vi "prop_axes_page_to_prop.vi"(10 "Axes Property Page":T1(array[cluster])) -> (2 "Axes Properties Out":T2)   [LabVIEW 2020, in "3DPC_SurfacePlot.xctl"]
uses:
  <vilib>/Native 3D Graph/xcontrol/3DPC_SurfacePlot.xctl
  <vilib>/Native 3D Graph/typedefs/prop_axes_all.ctl
  <vilib>/Native 3D Graph/typedefs/prop_axes_grid.ctl
  <vilib>/Native 3D Graph/typedefs/prop_axes_ticks.ctl
  <vilib>/Native 3D Graph/typedefs/range_cluster.ctl
  <vilib>/Native 3D Graph/typedefs/min_max.ctl
  <vilib>/Native 3D Graph/typedefs/prop_axes_captions.ctl
  <vilib>/Native 3D Graph/typedefs/prop_axes_labels.ctl
  <vilib>/Native 3D Graph/typedefs/prop_axes_autorange.ctl
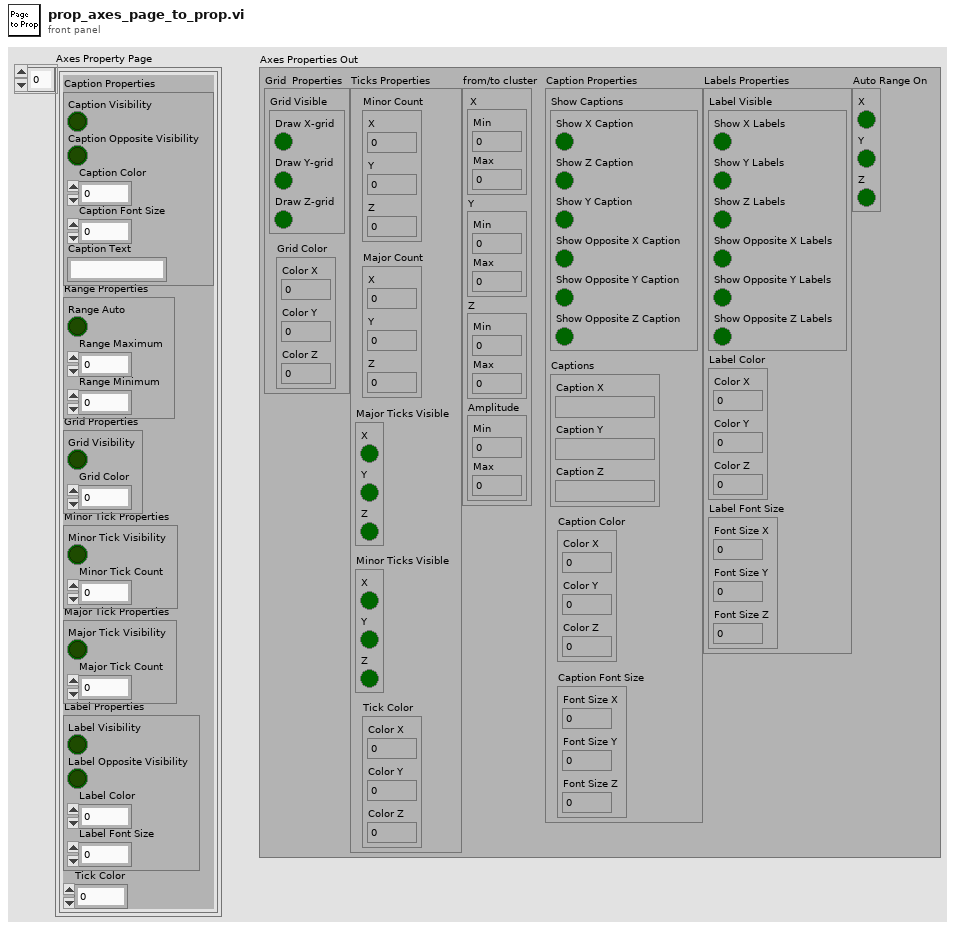
[diagram p1: front panel]
types:
  T1 = cluster{"Caption Properties":cluster{"Caption Visibility":bool, "Caption Opposite Visibility":bool, "Caption Color":u32, "Caption Font Size":i32, "Caption Text":string}, "Range Properties":cluster{"Range Auto":bool, "Range Maximum":dbl, "Range Minimum":dbl}, "Grid Properties":cluster{"Grid Visibility":bool, "Grid Color":u32}, "Minor Tick Properties":cluster{"Minor Tick Visibility":bool, "Minor Tick Count":i32}, "Major Tick Properties":cluster{"Major Tick Visibility":bool, "Major Tick Count":i32}, "Label Properties":cluster{"Label Visibility":bool, "Label Opposite Visibility":bool, "Label Color":u32, "Label Font Size":i32}, "Tick Color":u32}[]
  T2 = typedef "3DPC_SurfacePlot.xctl/prop_axes_all.ctl" = cluster{"Grid  Properties":T3, "Ticks Properties":T4, "from/to cluster":T5, "Caption Properties":T7, "Labels Properties":T8, "Auto Range On":T9}
  T3 = typedef "3DPC_SurfacePlot.xctl/prop_axes_grid.ctl" = cluster{"Grid Visible":cluster{"Draw X-grid":bool, "Draw Y-grid":bool, "Draw Z-grid":bool}, "Grid Color":cluster{"Color X":u32, "Color Y":u32, "Color Z":u32}}
  T4 = typedef "3DPC_SurfacePlot.xctl/prop_axes_ticks.ctl" = cluster{"Minor Count":cluster{"X":i32, "Y":i32, "Z":i32}, "Major Count":cluster{"X":i32, "Y":i32, "Z":i32}, "Major Ticks Visible":cluster{"X":bool, "Y":bool, "Z":bool}, "Minor Ticks Visible":cluster{"X":bool, "Y":bool, "Z":bool}, "Tick Color":cluster{"Color X":u32, "Color Y":u32, "Color Z":u32}}
  T5 = typedef "3DPC_SurfacePlot.xctl/range_cluster.ctl" = cluster{"X":T6, "Y":T6, "Z":T6, "Amplitude":T6}
  T6 = typedef "3DPC_SurfacePlot.xctl/min_max.ctl" = cluster{"Min":sgl, "Max":sgl}
  T7 = typedef "3DPC_SurfacePlot.xctl/prop_axes_captions.ctl" = cluster{"Show Captions":cluster{"Show X Caption":bool, "Show Z Caption":bool, "Show Y Caption":bool, "Show Opposite X Caption":bool, "Show Opposite Y Caption":bool, "Show Opposite Z Caption":bool}, "Captions":cluster{"Caption X":string, "Caption Y":string, "Caption Z":string}, "Caption Color":cluster{"Color X":u32, "Color Y":u32, "Color Z":u32}, "Caption Font Size":cluster{"Font Size X":i16, "Font Size Y":i16, "Font Size Z":i16}}
  T8 = typedef "3DPC_SurfacePlot.xctl/prop_axes_labels.ctl" = cluster{"Label Visible":cluster{"Show X Labels":bool, "Show Y Labels":bool, "Show Z Labels":bool, "Show Opposite X Labels":bool, "Show Opposite Y Labels":bool, "Show Opposite Z Labels":bool}, "Label Color":cluster{"Color X":u32, "Color Y":u32, "Color Z":u32}, "Label Font Size":cluster{"Font Size X":i16, "Font Size Y":i16, "Font Size Z":i16}}
  T9 = typedef "3DPC_SurfacePlot.xctl/prop_axes_autorange.ctl" = cluster{"X":bool, "Y":bool, "Z":bool}
  T10 = cluster{"Caption Properties":cluster{"Caption Visibility":bool, "Caption Opposite Visibility":bool, "Caption Color":u32, "Caption Font Size":i32, "Caption Text":string}, "Range Properties":cluster{"Range Auto":bool, "Range Maximum":dbl, "Range Minimum":dbl}, "Grid Properties":cluster{"Grid Visibility":bool, "Grid Color":u32}, "Minor Tick Properties":cluster{"Minor Tick Visibility":bool, "Minor Tick Count":i32}, "Major Tick Properties":cluster{"Major Tick Visibility":bool, "Major Tick Count":i32}, "Label Properties":cluster{"Label Visibility":bool, "Label Opposite Visibility":bool, "Label Color":u32, "Label Font Size":i32}, "Tick Color":u32}
  T11 = cluster{"Range Minimum":dbl, "Range Maximum":dbl}
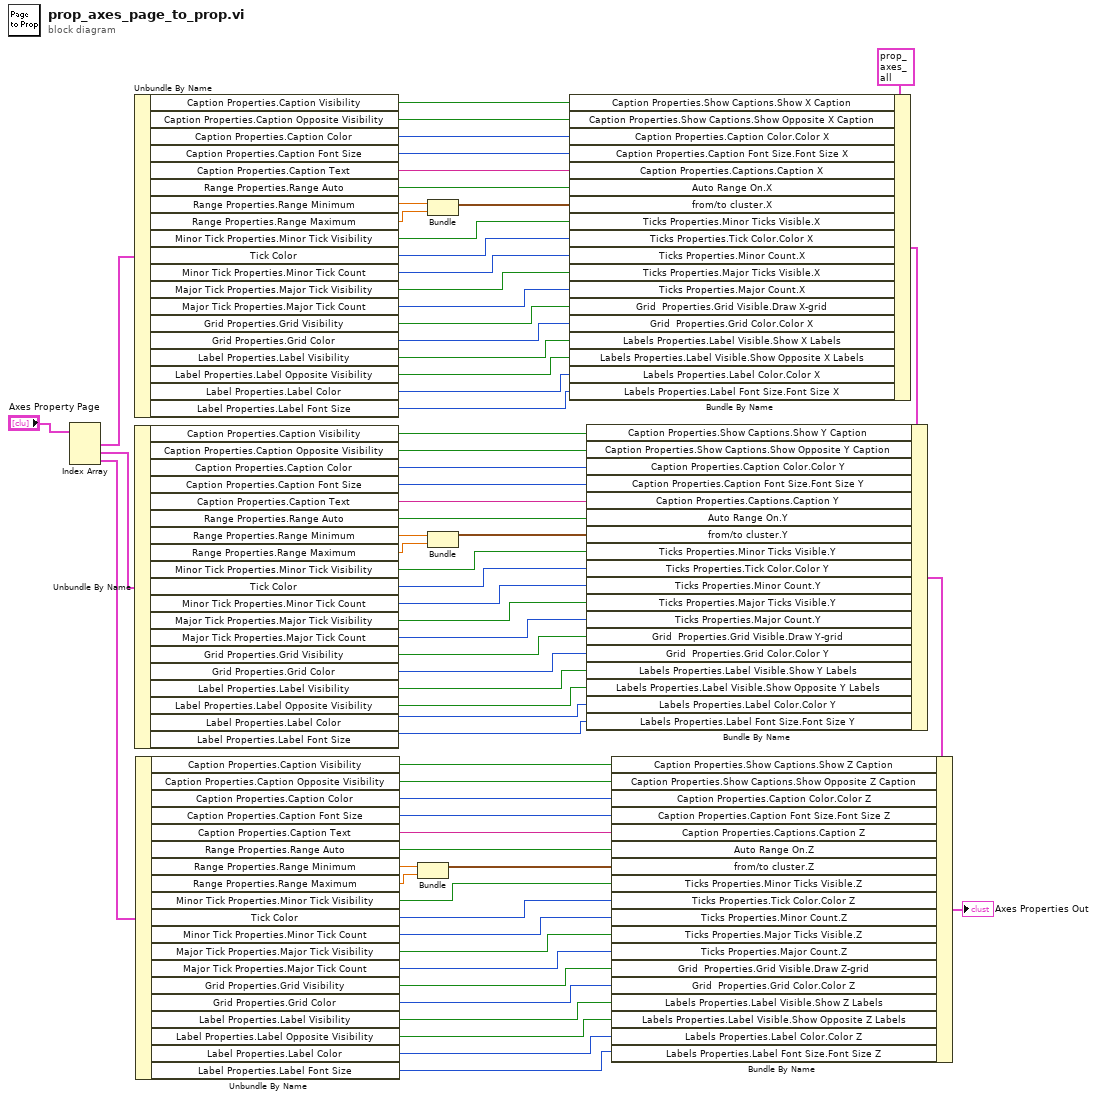
[diagram p0: block diagram]
diagram:
  n1 = Index Array(array="Axes Property Page") -> (element #1=w68:T10, element #2=w67:T10, element #3=w66:T10)  [unwired: 3 in]
  n2 = Unbundle By Name(w68) -> ("Caption Properties.Caption Visibility"=w58:bool, "Caption Properties.Caption Opposite Visibility"=w9:bool, "Caption Properties.Caption Color"=w57:u32, "Caption Properties.Caption Font Size"=w56:i32, "Caption Properties.Caption Text"=w55:string, "Range Properties.Range Auto"=w44:bool, "Range Properties.Range Minimum"=w65:dbl, "Range Properties.Range Maximum"=w64:dbl, "Minor Tick Properties.Minor Tick Visibility"=w54:bool, "Tick Color"=w53:u32, "Minor Tick Properties.Minor Tick Count"=w52:i32, "Major Tick Properties.Major Tick Visibility"=w51:bool, "Major Tick Properties.Major Tick Count"=w50:i32, "Grid Properties.Grid Visibility"=w49:bool, "Grid Properties.Grid Color"=w48:u32, "Label Properties.Label Visibility"=w47:bool, "Label Properties.Label Opposite Visibility"=w46:bool, "Label Properties.Label Color"=w45:u32, "Label Properties.Label Font Size"=w6:i32)
  n3 = Unbundle By Name(w67) -> ("Caption Properties.Caption Visibility"=w43:bool, "Caption Properties.Caption Opposite Visibility"=w8:bool, "Caption Properties.Caption Color"=w42:u32, "Caption Properties.Caption Font Size"=w41:i32, "Caption Properties.Caption Text"=w40:string, "Range Properties.Range Auto"=w39:bool, "Range Properties.Range Minimum"=w60:dbl, "Range Properties.Range Maximum"=w59:dbl, "Minor Tick Properties.Minor Tick Visibility"=w37:bool, "Tick Color"=w36:u32, "Minor Tick Properties.Minor Tick Count"=w35:i32, "Major Tick Properties.Major Tick Visibility"=w34:bool, "Major Tick Properties.Major Tick Count"=w33:i32, "Grid Properties.Grid Visibility"=w31:bool, "Grid Properties.Grid Color"=w30:u32, "Label Properties.Label Visibility"=w29:bool, "Label Properties.Label Opposite Visibility"=w28:bool, "Label Properties.Label Color"=w27:u32, "Label Properties.Label Font Size"=w5:i32)
  n4 = Unbundle By Name(w66) -> ("Caption Properties.Caption Visibility"=w25:bool, "Caption Properties.Caption Opposite Visibility"=w7:bool, "Caption Properties.Caption Color"=w24:u32, "Caption Properties.Caption Font Size"=w23:i32, "Caption Properties.Caption Text"=w22:string, "Range Properties.Range Auto"=w20:bool, "Range Properties.Range Minimum"=w62:dbl, "Range Properties.Range Maximum"=w61:dbl, "Minor Tick Properties.Minor Tick Visibility"=w19:bool, "Tick Color"=w2:u32, "Minor Tick Properties.Minor Tick Count"=w18:i32, "Major Tick Properties.Major Tick Visibility"=w17:bool, "Major Tick Properties.Major Tick Count"=w16:i32, "Grid Properties.Grid Visibility"=w15:bool, "Grid Properties.Grid Color"=w14:u32, "Label Properties.Label Visibility"=w13:bool, "Label Properties.Label Opposite Visibility"=w12:bool, "Label Properties.Label Color"=w11:u32, "Label Properties.Label Font Size"=w1:i32)
  n5 = Bundle("Range Minimum"=w62, "Range Maximum"=w61) -> (w21:T11)  [unwired: 1 out]
  n6 = Bundle("Range Minimum"=w65, "Range Maximum"=w64) -> (w63:T11)  [unwired: 1 out]
  n7 = Bundle("Range Minimum"=w60, "Range Maximum"=w59) -> (w38:T11)  [unwired: 1 out]
  n8 = Bundle By Name(cluster=T2 {"Grid  Properties"={"Grid Visible"={"Draw X-grid"=FALSE, "Draw Y-grid"=FALSE, "Draw Z-grid"=FALSE}, "Grid Color"={"Color X"=0, "Color Y"=0, "Color Z"=0}}, "Ticks Properties"={"Minor Count"={"X"=0, "Y"=0, "Z"=0}, "Major Count"={"X"=0, "Y"=0, "Z"=0}, "Major Ticks Visible"={"X"=FALSE, "Y"=FALSE, "Z"=FALSE}, "Minor Ticks Visible"={"X"=FALSE, "Y"=FALSE, "Z"=FALSE}, "Tick Color"={"Color X"=0, "Color Y"=0, "Color Z"=0}}, "from/to cluster"={"X"={"Min"=0.0, "Max"=0.0}, "Y"={"Min"=0.0, "Max"=0.0}, "Z"={"Min"=0.0, "Max"=0.0}, "Amplitude"={"Min"=0.0, "Max"=0.0}}, "Caption Properties"={"Show Captions"={"Show X Caption"=FALSE, "Show Z Caption"=FALSE, "Show Y Caption"=FALSE, "Show Opposite X Caption"=FALSE, "Show Opposite Y Caption"=FALSE, "Show Opposite Z Caption"=FALSE}, "Captions"={"Caption X"="", "Caption Y"="", "Caption Z"=""}, "Caption Color"={"Color X"=0, "Color Y"=0, "Color Z"=0}, "Caption Font Size"={"Font Size X"=0, "Font Size Y"=0, "Font Size Z"=0}}, "Labels Properties"={"Label Visible"={"Show X Labels"=FALSE, "Show Y Labels"=FALSE, "Show Z Labels"=FALSE, "Show Opposite X Labels"=FALSE, "Show Opposite Y Labels"=FALSE, "Show Opposite Z Labels"=FALSE}, "Label Color"={"Color X"=0, "Color Y"=0, "Color Z"=0}, "Label Font Size"={"Font Size X"=0, "Font Size Y"=0, "Font Size Z"=0}}, "Auto Range On"={"X"=FALSE, "Y"=FALSE, "Z"=FALSE}} ("Axes Properties"), "Caption Properties.Show Captions.Show X Caption"=w58, "Caption Properties.Show Captions.Show Opposite X Caption"=w9, "Caption Properties.Caption Color.Color X"=w57, "Caption Properties.Caption Font Size.Font Size X"=w56, "Caption Properties.Captions.Caption X"=w55, "Auto Range On.X"=w44, "from/to cluster.X"=w63, "Ticks Properties.Minor Ticks Visible.X"=w54, "Ticks Properties.Tick Color.Color X"=w53, "Ticks Properties.Minor Count.X"=w52, "Ticks Properties.Major Ticks Visible.X"=w51, "Ticks Properties.Major Count.X"=w50, "Grid  Properties.Grid Visible.Draw X-grid"=w49, "Grid  Properties.Grid Color.Color X"=w48, "Labels Properties.Label Visible.Show X Labels"=w47, "Labels Properties.Label Visible.Show Opposite X Labels"=w46, "Labels Properties.Label Color.Color X"=w45, "Labels Properties.Label Font Size.Font Size X"=w6) -> (w32:T2)
  n9 = Bundle By Name(cluster=w32, "Caption Properties.Show Captions.Show Y Caption"=w43, "Caption Properties.Show Captions.Show Opposite Y Caption"=w8, "Caption Properties.Caption Color.Color Y"=w42, "Caption Properties.Caption Font Size.Font Size Y"=w41, "Caption Properties.Captions.Caption Y"=w40, "Auto Range On.Y"=w39, "from/to cluster.Y"=w38, "Ticks Properties.Minor Ticks Visible.Y"=w37, "Ticks Properties.Tick Color.Color Y"=w36, "Ticks Properties.Minor Count.Y"=w35, "Ticks Properties.Major Ticks Visible.Y"=w34, "Ticks Properties.Major Count.Y"=w33, "Grid  Properties.Grid Visible.Draw Y-grid"=w31, "Grid  Properties.Grid Color.Color Y"=w30, "Labels Properties.Label Visible.Show Y Labels"=w29, "Labels Properties.Label Visible.Show Opposite Y Labels"=w28, "Labels Properties.Label Color.Color Y"=w27, "Labels Properties.Label Font Size.Font Size Y"=w5) -> (w26:T2)
  n10 = Bundle By Name(cluster=w26, "Caption Properties.Show Captions.Show Z Caption"=w25, "Caption Properties.Show Captions.Show Opposite Z Caption"=w7, "Caption Properties.Caption Color.Color Z"=w24, "Caption Properties.Caption Font Size.Font Size Z"=w23, "Caption Properties.Captions.Caption Z"=w22, "Auto Range On.Z"=w20, "from/to cluster.Z"=w21, "Ticks Properties.Minor Ticks Visible.Z"=w19, "Ticks Properties.Tick Color.Color Z"=w2, "Ticks Properties.Minor Count.Z"=w18, "Ticks Properties.Major Ticks Visible.Z"=w17, "Ticks Properties.Major Count.Z"=w16, "Grid  Properties.Grid Visible.Draw Z-grid"=w15, "Grid  Properties.Grid Color.Color Z"=w14, "Labels Properties.Label Visible.Show Z Labels"=w13, "Labels Properties.Label Visible.Show Opposite Z Labels"=w12, "Labels Properties.Label Color.Color Z"=w11, "Labels Properties.Label Font Size.Font Size Z"=w1) -> (→"Axes Properties Out":T2)
